vi "Actor Core.vi"(8 "error in":errorcluster, 11 "Nested in":refnum<class "Mensajes.lvclass">) -> (0 "error out":errorcluster, 3 "Actor out":refnum<class "Actor.lvclass">)   [LabVIEW 2021, in "Mensajes.lvlib" / "Mensajes.lvclass"]
doc: "(<B>Filename</B>: Actor Framework.lvlib:Actor.lvclass:Actor Core.vi)\n\nReceives messages to the actor, reacts to them, and initiates any error handling that may shut the actor down.\n\nDescendant classes may override this VI to append parallel tasks for the actor to complete while it handles messages. Overrides use the Call Parent Method node."
uses:
  Mensajes.lvclass
  C:/Program Files (x86)/National Instruments/LabVIEW 2021/vi.lib/ActorFramework/Actor/Actor.lvclass
  <vilib>/ActorFramework/Actor/Actor.lvclass
  <vilib>/ActorFramework/Actor/Actor.lvclass/Actor.ctl
  <vilib>/ActorFramework/Message Enqueuer/Message Enqueuer.lvclass/Message Enqueuer.ctl
  Mensajes.lvclass/Mensajes.ctl
  <vilib>/ActorFramework/Message Enqueuer/Init from Existing Queue.vi
  <vilib>/ActorFramework/Message Enqueuer/Enqueue.vi
  <vilib>/ActorFramework/Stop Msg/Stop Msg.lvclass
  C:/Program Files (x86)/National Instruments/LabVIEW 2021/vi.lib/ActorFramework/Message/Message.lvclass
  <vilib>/ActorFramework/Message Priority Queue/Priority Enqueue.vi
  <vilib>/ActorFramework/Message Enqueuer/Message Enqueuer.lvclass
  C:/Users/scrap/Fork/Vending Machine AF/Actor-Framework-Vending-Machine/Vending Machine AF Folder/Mensajes/Mensajes.lvclass
panel:
  out "Status":string
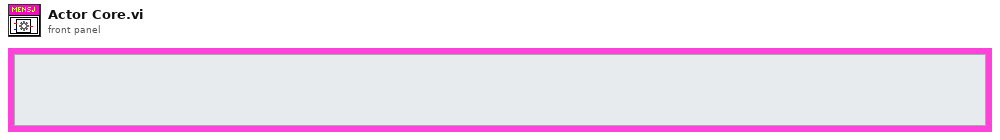
[diagram p1: front panel]
types:
  T1 = cluster{"Stop":refnum<user-event>, "Status":refnum<user-event>}
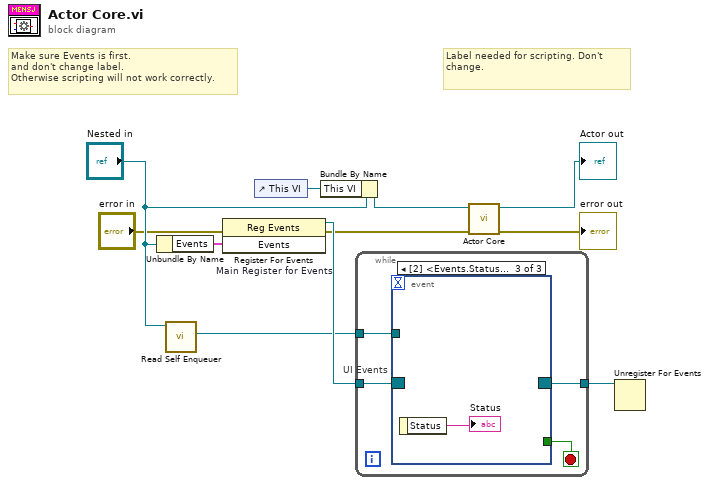
[diagram p0: block diagram]
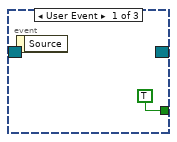
[diagram p2: hidden frame]
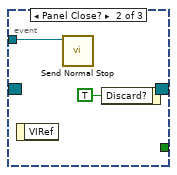
[diagram p3: hidden frame]
diagram:
  # "Label needed for scripting. Don't change."
  # "Make sure Events is first.\nand don't change label.\nOtherwise scripting will not work correctly."
  n1 = Unbundle By Name("Nested in") -> ("Events"=w8:T1)
  n2 = call <vilib>:"Read Self Enqueuer.vi"("Actor"="Nested in") -> ("Self Enqueuer"=w5:refnum<class "Message Enqueuer.lvclass">)  [unwired: 10 in]
  n3 = register-events "Main Register for Events"(error in="error in", w8) -> (reference out=w9:refnum<event-registration>, error out=w3:errorcluster)  [unwired: 1 in]
  n4 = control-ref of="This VI"() -> (w1:refnum<vi>)
  n5 = Bundle By Name(cluster="Nested in", "This VI"=w1) -> (w2:refnum<class "Mensajes.lvclass">)
  n6 = while {
    tunnel: w9 -> [w15]
    tunnel: [w13] -> w7
    tunnel: w5 -> [w12]
    stop <- w14 stop-if-true
    n7 = event "UI Events" shown="[2] <Events.Status>: User Event" {
      selector: w15 -> [_ _ _]
      dyn-events: [_ _ _] -> w13
      timeout: _ -> [_ _ _]
      tunnel: [TRUE _ _] -> w14
      tunnel: w12 -> [_ w17 _]
      event User Event {
        n8 = event-data() -> ()  [unwired: 1 in, 1 out]
      }
      event Panel Close? {
        n9 = event-data() -> ()  [unwired: 1 in, 1 out]
        n10 = call <vilib>:"Send Normal Stop.vi"("Message Enqueuer"=w17) -> ()  [unwired: 10 in, 1 out]
        n11 = event-data("Discard?"=TRUE) -> ()  [unwired: 1 in, 1 out]
      }
      event User Event {
        n12 = event-data() -> ("Status"=→"Status":string)  [unwired: 1 in]
      }
    }
  }
  n13 = call-parent "Actor Core.vi"("error in"=w3, "Actor in"=w2) -> ("error out"=→"error out":errorcluster, "Actor out"=→"Actor out":refnum<class "Actor.lvclass">)  [unwired: 8 in]
  n14 = Unregister For Events(event registration refnum=w7) -> ()  [unwired: 1 in, 1 out]
